vi "acquireValue.vi"(8 "error in (no error)":errorcluster, 10 "nextSample?":bool, 11 "enterControl in":refnum<class "enterControl.lvclass">) -> (0 "error out":errorcluster, 1 "function return":i32, 2 "variantData":variant, 3 "enterControl out":refnum<class "enterControl.lvclass">)   [LabVIEW 2016, in "SALLV_EXA_Messaging.lvlib" / "enterControl.lvclass"]
uses:
  enterControl.lvclass
  enterControl.lvclass/enterControl.ctl
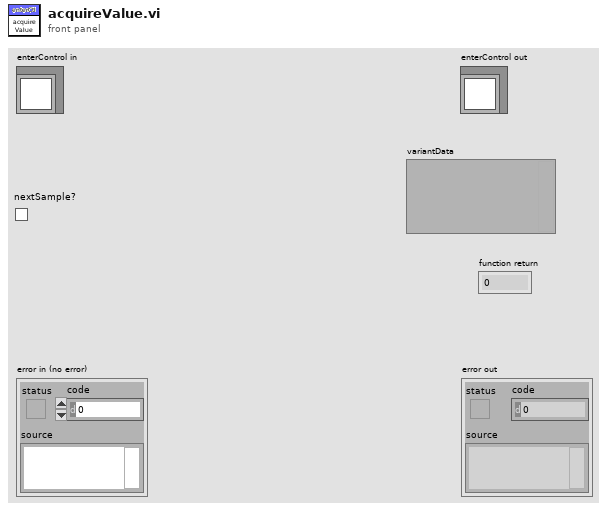
[diagram p1: front panel]
types:
  T1 = typedef "SALLV_EXA.lvlib/command_disable.ctl" = cluster{"value":bool}
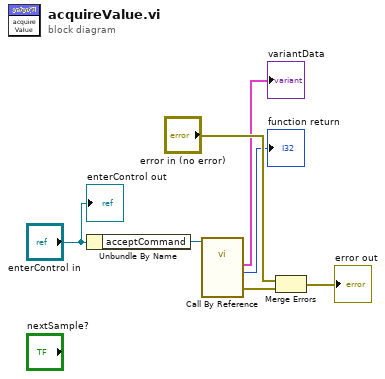
[diagram p0: block diagram]
diagram:
  n1 = Unbundle By Name("enterControl in") -> ("acceptCommand"=w6:refnum<vi>)
  n2 = call-by-ref "?"(reference=w6) -> ("error out"=w7:errorcluster, "function return"=→"function return":i32, "command_disable_Ctl out"=→"variantData":T1)  [unwired: 10 in, 2 out]
  n3 = Merge Errors("error in (no error)", w7) -> (→"error out":errorcluster)
  "enterControl out" <- "enterControl in"
